vi "GetPubs.vi"(8 "error in (no error)":errorcluster, 11 "S4GUI in":refnum<class "S4GUI.lvclass">) -> (0 "error out":errorcluster, 2 "Pubs out":T1, 3 "S4GUI out":refnum<class "S4GUI.lvclass">)   [LabVIEW 2018, in "S4GUI.lvclass"]
uses:
  S4GUI.lvclass
  S4GUI.lvclass/S4GUI.ctl
  Publisher/Publisher.lvclass
  Acquisition/Acquisition.lvclass
  Instrument/Instrument.lvclass
  TCS/TCS.lvclass
  TelFocus/TelFocus.lvclass
  WeatherStation/WeatherStation.lvclass
  GSserver/GSserver.lvclass
  Comm/Stream/Stream.lvclass
panel:
  out "lastPub":string
  in  "Pubs":T1
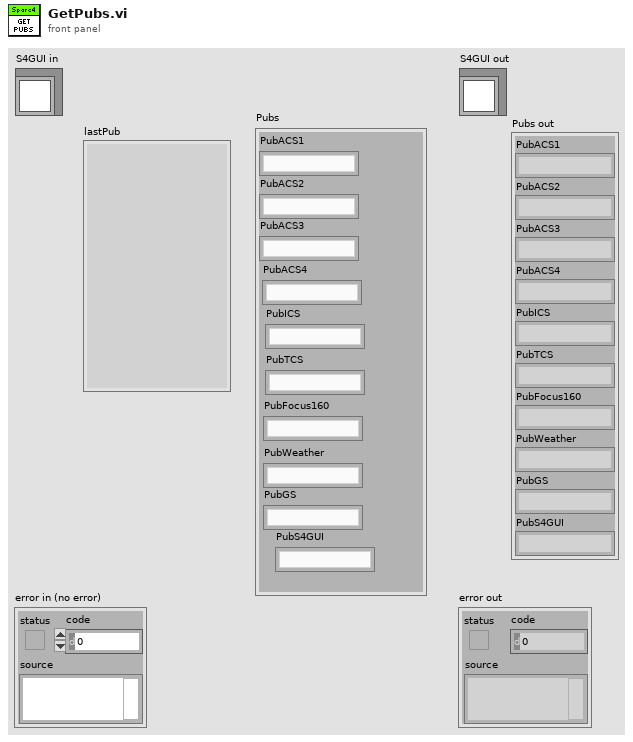
[diagram p1: front panel]
types:
  T1 = cluster{"PubACS1":string, "PubACS2":string, "PubACS3":string, "PubACS4":string, "PubICS":string, "PubTCS":string, "PubFocus160":string, "PubWeather":string, "PubGS":string, "PubS4GUI":string}
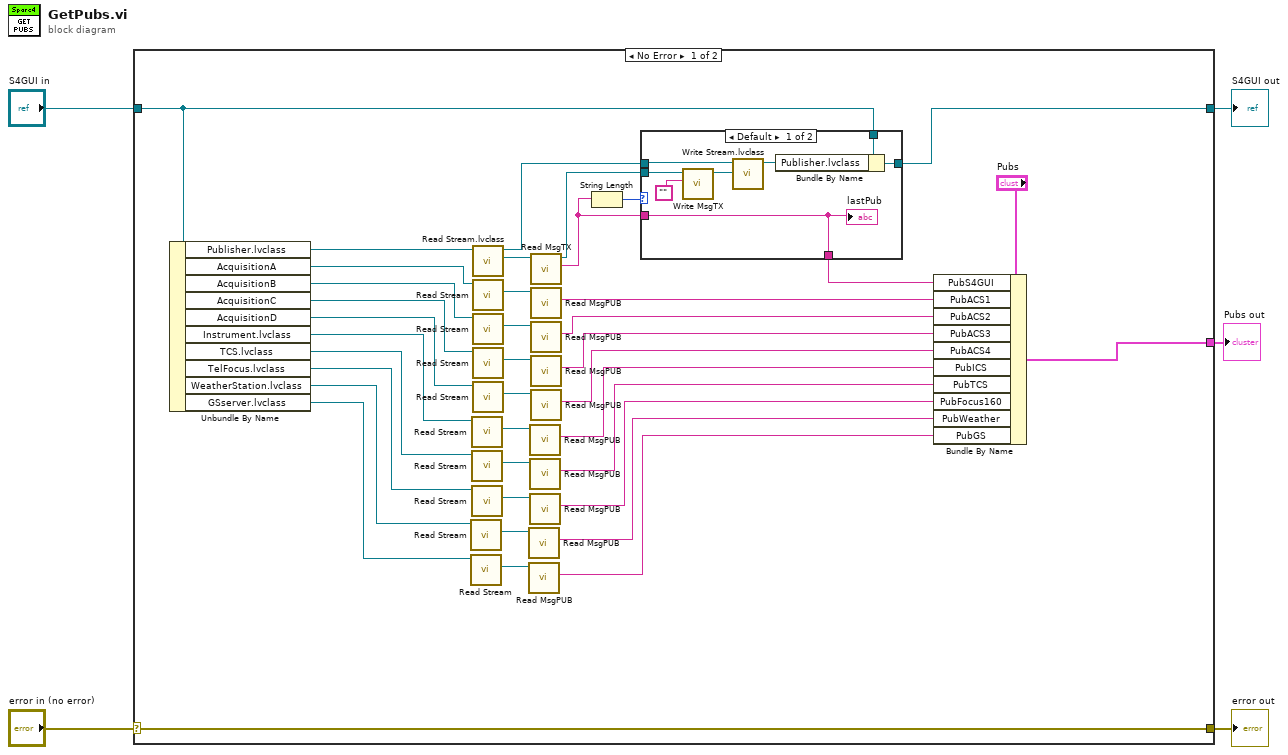
[diagram p0: block diagram]
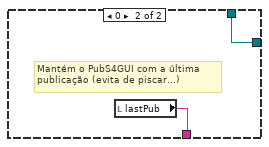
[diagram p2: hidden frame]
diagram:
  n1 = case shown="No Error" "error in (no error)" {
    selector: "error in (no error)" -> [w44 w56]
    tunnel: [w44 w56] -> w4
    tunnel: [w11 w55] -> w2
    tunnel: "S4GUI in" -> [w12 w55]
    tunnel: [w29 _] -> w1
    frame No Error {
      n2 = Unbundle By Name(w12) -> ("Publisher.lvclass"=w43:refnum<class "Publisher.lvclass">, "AcquisitionA"=w41:refnum<class "Acquisition.lvclass">, "AcquisitionB"=w38:refnum<class "Acquisition.lvclass">, "AcquisitionC"=w35:refnum<class "Acquisition.lvclass">, "AcquisitionD"=w32:refnum<class "Acquisition.lvclass">, "Instrument.lvclass"=w28:refnum<class "Instrument.lvclass">, "TCS.lvclass"=w25:refnum<class "TCS.lvclass">, "TelFocus.lvclass"=w22:refnum<class "TelFocus.lvclass">, "WeatherStation.lvclass"=w19:refnum<class "WeatherStation.lvclass">, "GSserver.lvclass"=w16:refnum<class "GSserver.lvclass">)
      n3 = call-dynamic "Read Stream.vi"("Server in"=w19) -> ("Stream.lvclass"=w18:refnum<class "Stream.lvclass">)  [unwired: 8 in, 2 out]
      n4 = call-dynamic "Read Stream.vi"("Server in"=w16) -> ("Stream.lvclass"=w15:refnum<class "Stream.lvclass">)  [unwired: 8 in, 2 out]
      n5 = call-dynamic "Read Stream.vi"("Server in"=w28) -> ("Stream.lvclass"=w27:refnum<class "Stream.lvclass">)  [unwired: 8 in, 2 out]
      n6 = call-dynamic "Read Stream.vi"("Server in"=w25) -> ("Stream.lvclass"=w24:refnum<class "Stream.lvclass">)  [unwired: 8 in, 2 out]
      n7 = call-dynamic "Read Stream.vi"("Server in"=w22) -> ("Stream.lvclass"=w21:refnum<class "Stream.lvclass">)  [unwired: 8 in, 2 out]
      n8 = call-dynamic "Read Stream.lvclass.vi"("Client in"=w43) -> ("Stream.lvclass"=w42:refnum<class "Stream.lvclass">, "Client out"=w10:refnum<class "Publisher.lvclass">)  [unwired: 8 in, 1 out]
      n9 = call-dynamic "Read Stream.vi"("Server in"=w41) -> ("Stream.lvclass"=w40:refnum<class "Stream.lvclass">)  [unwired: 8 in, 2 out]
      n10 = call-dynamic "Read Stream.vi"("Server in"=w38) -> ("Stream.lvclass"=w37:refnum<class "Stream.lvclass">)  [unwired: 8 in, 2 out]
      n11 = call-dynamic "Read Stream.vi"("Server in"=w35) -> ("Stream.lvclass"=w34:refnum<class "Stream.lvclass">)  [unwired: 8 in, 2 out]
      n12 = call-dynamic "Read Stream.vi"("Server in"=w32) -> ("Stream.lvclass"=w31:refnum<class "Stream.lvclass">)  [unwired: 8 in, 2 out]
      n13 = call-dynamic "Read MsgPUB.vi"("Comm in"=w18) -> ("MsgPUB"=w17:string)  [unwired: 8 in, 2 out]
      n14 = call-dynamic "Read MsgPUB.vi"("Comm in"=w15) -> ("MsgPUB"=w14:string)  [unwired: 8 in, 2 out]
      n15 = call-dynamic "Read MsgPUB.vi"("Comm in"=w27) -> ("MsgPUB"=w26:string)  [unwired: 8 in, 2 out]
      n16 = call-dynamic "Read MsgPUB.vi"("Comm in"=w24) -> ("MsgPUB"=w23:string)  [unwired: 8 in, 2 out]
      n17 = call-dynamic "Read MsgPUB.vi"("Comm in"=w21) -> ("MsgPUB"=w20:string)  [unwired: 8 in, 2 out]
      n18 = call-dynamic "Read MsgTX.vi"("Comm in"=w42) -> ("MsgTX"=w8:string, "Comm out"=w13:refnum<class "Stream.lvclass">)  [unwired: 8 in, 1 out]
      n19 = call-dynamic "Read MsgPUB.vi"("Comm in"=w40) -> ("MsgPUB"=w39:string)  [unwired: 8 in, 2 out]
      n20 = call-dynamic "Read MsgPUB.vi"("Comm in"=w37) -> ("MsgPUB"=w36:string)  [unwired: 8 in, 2 out]
      n21 = call-dynamic "Read MsgPUB.vi"("Comm in"=w34) -> ("MsgPUB"=w33:string)  [unwired: 8 in, 2 out]
      n22 = call-dynamic "Read MsgPUB.vi"("Comm in"=w31) -> ("MsgPUB"=w30:string)  [unwired: 8 in, 2 out]
      n23 = String Length(string=w8) -> (length=w9:i32)
      n24 = case shown="Default" w9 {
        tunnel: w13 -> [w50 _]
        tunnel: w12 -> [w52 w54]
        tunnel: [w51 w54] -> w11
        tunnel: w10 -> [w49 _]
        tunnel: w8 -> [w45 _]
        tunnel: [w45 w53] -> w6
        frame Default {
          n25 = call-dynamic "Write MsgTX.vi"("MsgTX"="", "Comm in"=w50) -> ("Comm out"=w47:refnum<class "Stream.lvclass">)  [unwired: 8 in, 1 out]
          n26 = call-dynamic "Write Stream.lvclass.vi"("Stream.lvclass"=w47, "Client in"=w49) -> ("Client out"=w48:refnum<class "Publisher.lvclass">)  [unwired: 8 in, 1 out]
          n27 = Bundle By Name(cluster=w52, "Publisher.lvclass"=w48) -> (w51:refnum<class "S4GUI.lvclass">)
          "lastPub" <- w45
        }
        frame 0 {
          # "Mantém o PubS4GUI com a última\npublicação (evita de piscar...)"
          n28 = local read "lastPub"() -> (w53:string)
        }
      }
      n29 = Bundle By Name(cluster="Pubs", "PubS4GUI"=w6, "PubACS1"=w39, "PubACS2"=w36, "PubACS3"=w33, "PubACS4"=w30, "PubICS"=w26, "PubTCS"=w23, "PubFocus160"=w20, "PubWeather"=w17, "PubGS"=w14) -> (w29:T1)
    }
    frame Error {
    }
  }
  "error out" <- w4
  "S4GUI out" <- w2
  "Pubs out" <- w1
